vi "Write Sampling Rate Bits.vi"(8 "error in (no error)":errorcluster, 10 "Sampling Rate Bits":u16, 11 "LINX-ADS1X15 in":refnum<class "LINX-ADS1256.lvclass">) -> (0 "error out":errorcluster, 3 "LINX-ADS1X15 out":refnum<class "LINX-ADS1256.lvclass">)   [LabVIEW 2020, in "LINX-ADS1256.lvclass"]
uses:
  LINX-ADS1256.lvclass
  LINX-ADS1256.lvclass/LINX-ADS1256.ctl
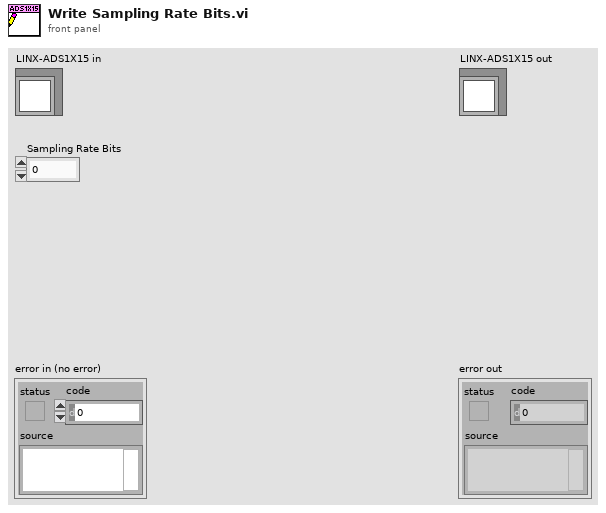
[diagram p1: front panel]
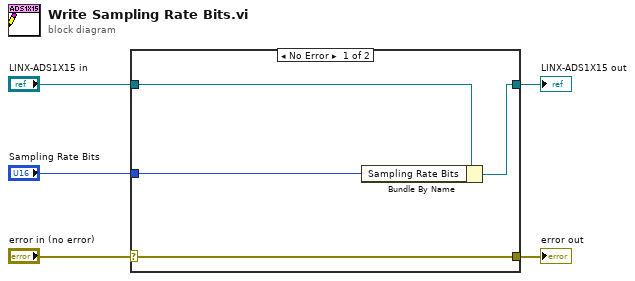
[diagram p0: block diagram]
diagram:
  n1 = case shown="No Error" "error in (no error)" {
    selector: "error in (no error)" -> [w9 w10]
    tunnel: [w9 w10] -> w4
    tunnel: [w7 w11] -> w2
    tunnel: "LINX-ADS1X15 in" -> [w8 w11]
    tunnel: "Sampling Rate Bits" -> [w6 _]
    frame No Error {
      n2 = Bundle By Name(cluster=w8, "Sampling Rate Bits"=w6) -> (w7:refnum<class "LINX-ADS1256.lvclass">)
    }
    frame Error {
    }
  }
  "error out" <- w4
  "LINX-ADS1X15 out" <- w2
